vi "GenNewTraj.vi"(4 "MEGA traj":T1 {"?"."Limits"."StoopidFast (fps)" min=0.0; "?"."Limits"."Jerk (fps^3)" min=0.0 step=1.0; "?"."Limits"."Accel (fps^2)" min=0.0; "?"."Limits"."Velocity (fps)" min=0.0; "?"."Overrides"."Angle Override" step=5.0; "?"."Overrides"."Velocity Override" step=5.0; "?"."Overrides"."Angular Override" step=5.0; "?"."Angular Limits"."Jerk (deg/s^3)" min=0.0 step=1.0; "?"."Angular Limits"."Accel (deg/s^2)" min=0.0; "?"."Angular Limits"."Velocity (deg/s)" min=0.0}, 6 "Drive Type":T9, 7 "MEGA?":bool, 8 "Stoopid Overlap %":dbl min=0.0, 9 "Path Type":T10, 10 "Parameters":T11 {"Limits"."StoopidFast (fps)" min=0.0; "Limits"."Jerk (fps^3)" min=0.0 step=1.0; "Limits"."Accel (fps^2)" min=0.0; "Limits"."Velocity (fps)" min=0.0; "Overrides"."Angle Override" step=5.0; "Overrides"."Velocity Override" step=5.0; "Overrides"."Angular Override" step=5.0; "Angular Limits"."Jerk (deg/s^3)" min=0.0 step=1.0; "Angular Limits"."Accel (deg/s^2)" min=0.0; "Angular Limits"."Velocity (deg/s)" min=0.0}, 11 "Points in":cluster{"x":dbl, "y":dbl, "th":dbl}[](array[cluster])) -> (0 "Time & Dist":cluster{"Time (s)":dbl, "Distance (ft)":dbl}, 1 "Valid":bool, 2 "Trajectory Data":T2, 3 "Updated Waypoints":cluster{"x":dbl, "y":dbl, "th":dbl}[](array[cluster]), 5 "MEGA traj 2":T1 {"?"."Limits"."StoopidFast (fps)" min=0.0; "?"."Limits"."Jerk (fps^3)" min=0.0 step=1.0; "?"."Limits"."Accel (fps^2)" min=0.0; "?"."Limits"."Velocity (fps)" min=0.0; "?"."Overrides"."Angle Override" step=5.0; "?"."Overrides"."Velocity Override" step=5.0; "?"."Overrides"."Angular Override" step=5.0; "?"."Angular Limits"."Jerk (deg/s^3)" min=0.0 step=1.0; "?"."Angular Limits"."Accel (deg/s^2)" min=0.0; "?"."Angular Limits"."Velocity (deg/s)" min=0.0})   [LabVIEW 2023]
uses:
  Types/Trajectory Data.ctl
  Types/Segment Type.ctl
  Types/Path Type.ctl
  Types/Limits.ctl
  Types/Overrides.ctl
  Types/Angluar Limits.ctl
  Types/Drive Type.ctl
  FileIO/MEGA traj.ctl
  Types/Single Cmd Info.ctl
  <vilib>/picture/picture.llb/imagedata.ctl
  Bezier/Bezier Trajectory.vi
  Clothoid/Generate Clothoid Trajectory.vi
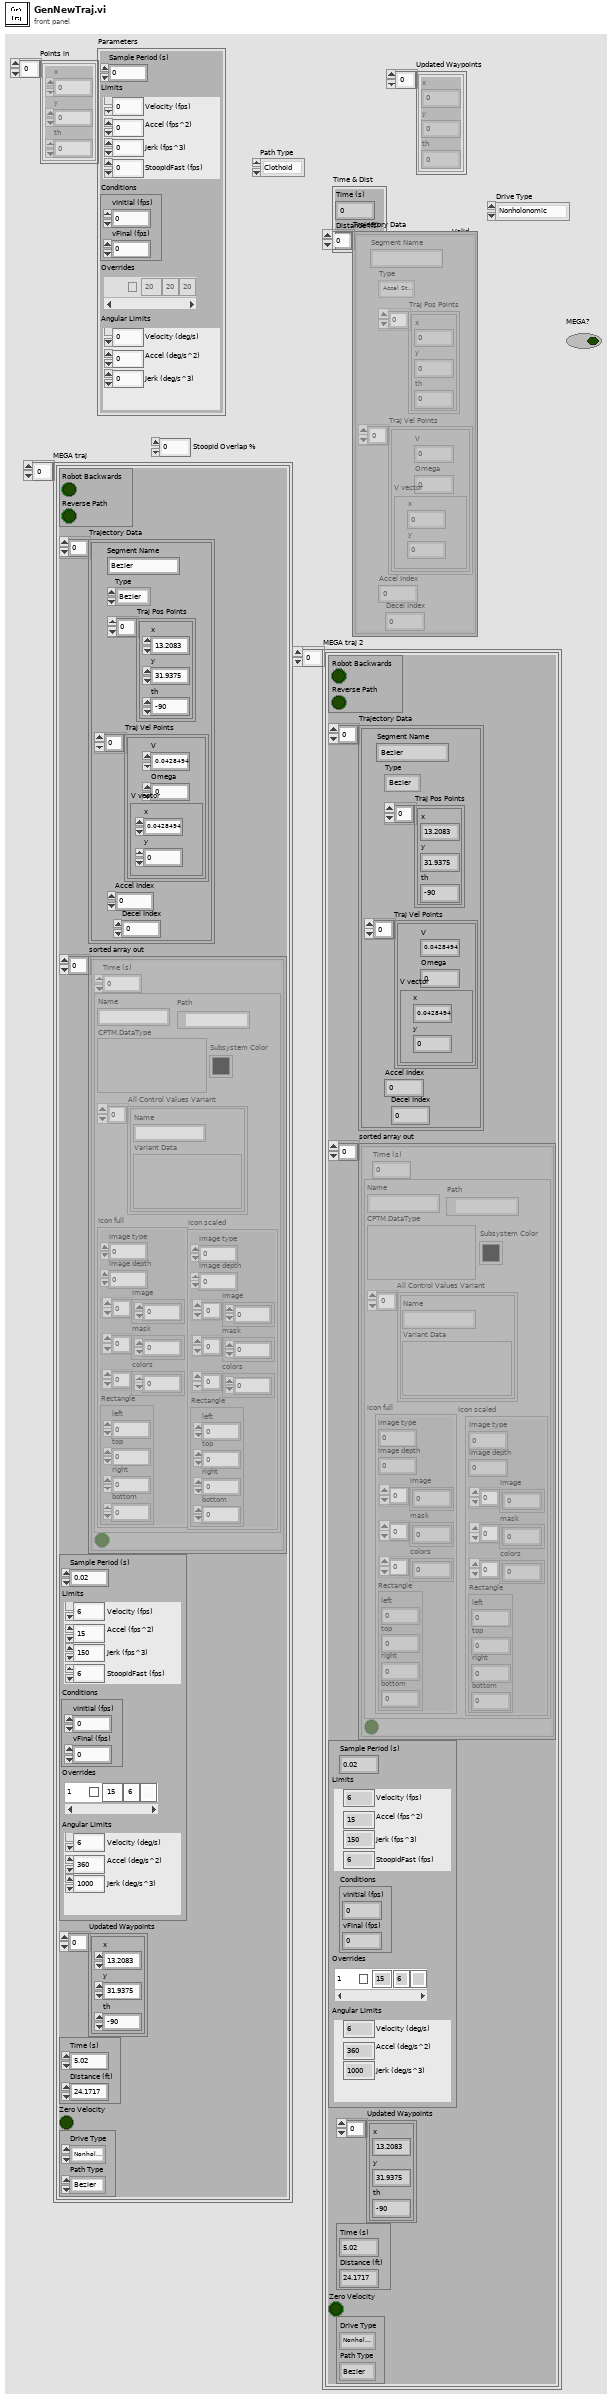
[diagram p1: front panel]
types:
  T1 = typedef "MEGA traj.ctl" = cluster{cluster{"Robot Backwards":bool, "Reverse Path":bool}, "Trajectory Data":T2, "sorted array out":cluster{"Time (s)":dbl, T4, bool}[], cluster{"Sample Period (s)":dbl, "Limits":T6, "Conditions":cluster{"vInitial (fps)":dbl, "vFinal (fps)":dbl}, "Overrides":T7, "Angular Limits":T8}, "Updated Waypoints":cluster{"x":dbl, "y":dbl, "th":dbl}[], cluster{"Time (s)":dbl, "Distance (ft)":dbl}, "Zero Velocity":bool, cluster{"Drive Type":T9, "Path Type":T10}}[]
  T2 = typedef "Trajectory Data.ctl" = cluster{"Segment Name":string, "Type":T3, "Traj Pos Points":cluster{"x":dbl, "y":dbl, "th":dbl}[], "Traj Vel Points":cluster{"V":dbl, "Omega":dbl, "V vector":cluster{"y":dbl, "x":dbl}}[], "Accel Index":i32, "Decel Index":i32}[]
  T3 = typedef "Segment Type.ctl" = enum16{"Accel Straight", "Const Straight", "Blend", "Circle", "Bezier"}
  T4 = typedef "Single Cmd Info.ctl" = cluster{"Name":string, "CPTM.DataType":variant, "All Control Values Variant":cluster{"Name":string, "Variant Data":variant}[], "icon full":T5, "icon scaled":T5, "Path":path, "Subsystem Color":u32}
  T5 = typedef "imagedata.ctl" = cluster{"image type":i32, "image depth":i32, "image":u8[], "mask":u8[], "colors":u32[], "Rectangle":cluster{"left":i16, "top":i16, "right":i16, "bottom":i16}}
  T6 = typedef "Limits.ctl" = cluster{"Velocity (fps)":dbl, "Accel (fps^2)":dbl, "Jerk (fps^3)":dbl, "StoopidFast (fps)":dbl}
  T7 = typedef "Overrides.ctl" = cluster{"Count":string, "Angular Override":dbl, "Enabled?":bool, "Velocity Override":dbl, "Angle Override":dbl}[]
  T8 = typedef "Angluar Limits.ctl" = cluster{"Velocity (deg/s)":dbl, "Accel (deg/s^2)":dbl, "Jerk (deg/s^3)":dbl}
  T9 = typedef "Drive Type.ctl" = enum16{"Nonholonomic", "Holonomic"}
  T10 = typedef "Path Type.ctl" = enum16{"Clothoid", "Bezier"}
  T11 = cluster{"Sample Period (s)":dbl, "Limits":T6, "Conditions":cluster{"vInitial (fps)":dbl, "vFinal (fps)":dbl}, "Overrides":T7, "Angular Limits":T8}
  T12 = cluster{"Robot Backwards":bool, "Reverse Path":bool}
  T13 = cluster{"vInitial (fps)":dbl, "vFinal (fps)":dbl}
  T14 = cluster{"Segment Name":string, "Type":T3, "Traj Pos Points":cluster{"x":dbl, "y":dbl, "th":dbl}[], "Traj Vel Points":cluster{"V":dbl, "Omega":dbl, "V vector":cluster{"y":dbl, "x":dbl}}[], "Accel Index":i32, "Decel Index":i32}[]
  T15 = cluster{cluster{"Robot Backwards":bool, "Reverse Path":bool}, "Trajectory Data":T2, "sorted array out":cluster{"Time (s)":dbl, T4, bool}[], cluster{"Sample Period (s)":dbl, "Limits":T6, "Conditions":cluster{"vInitial (fps)":dbl, "vFinal (fps)":dbl}, "Overrides":T7, "Angular Limits":T8}, "Updated Waypoints":cluster{"x":dbl, "y":dbl, "th":dbl}[], cluster{"Time (s)":dbl, "Distance (ft)":dbl}, "Zero Velocity":bool, cluster{"Drive Type":T9, "Path Type":T10}}
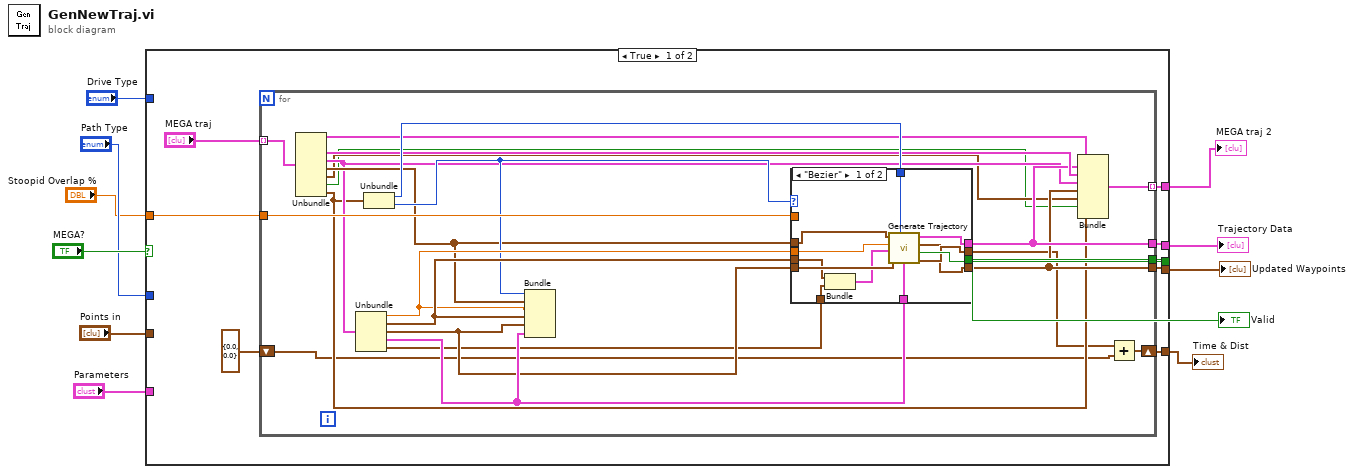
[diagram p0: block diagram]
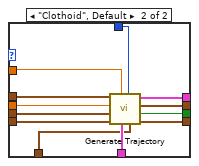
[diagram p2: hidden frame]
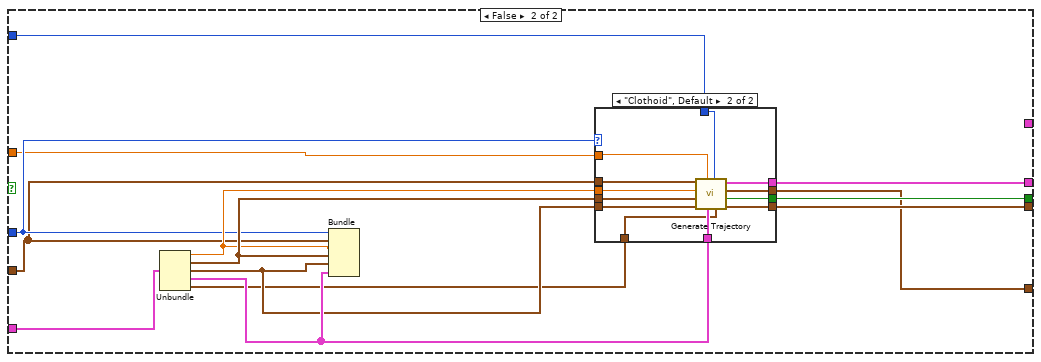
[diagram p3: hidden frame]
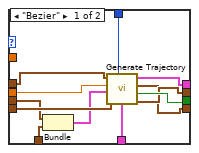
[diagram p4: hidden frame]
diagram:
  n1 = case shown="True" "MEGA?" {
    tunnel: [w17 w80] -> w11
    tunnel: [w16 w79] -> w10
    tunnel: [w18 w75] -> w9
    tunnel: [w19 w73] -> w8
    tunnel: "Drive Type" -> [_ w71]
    tunnel: "Path Type" -> [_ w70]
    tunnel: "Stoopid Overlap %" -> [w14 w69]
    tunnel: "Points in" -> [_ w68]
    tunnel: "Parameters" -> [_ w67]
    tunnel: [w13 _] -> w1
    frame True {
      n2 = for {
        tunnel: [w29] -> w19
        tunnel: [w37] -> w17
        tunnel: [w27] -> w16
        tunnel: w14 -> [w36]
        tunnel: "MEGA traj" -> [w35] mode=indexing
        tunnel: [w23] -> w13 mode=indexing
        shift-right: [w22] -> w18
        shift-left: cluster{"Time (s)":dbl, "Distance (ft)":dbl} {"Time (s)"=0.0, "Distance (ft)"=0.0} -> [w20]
        n3 = Unbundle(w35) -> (w31:T12, "sorted array out"=w30:cluster{"Time (s)":dbl, T4, bool}[], w28:T11, "Updated Waypoints"=w32:cluster{"x":dbl, "y":dbl, "th":dbl}[], w26:cluster{"Time (s)":dbl, "Distance (ft)":dbl}, "Zero Velocity"=w25:bool, w24:cluster{"Drive Type":T9, "Path Type":T10})  [unwired: 1 out]
        n4 = Unbundle(w28) -> ("Sample Period (s)"=w39:dbl, "Limits"=w41:T6, "Conditions"=w40:T13, "Overrides"=w42:T7, "Angular Limits"=w38:T8)
        n5 = Unbundle(w24) -> ("Drive Type"=w34:T9, "Path Type"=w33:T10)
        n6 = Bundle("Path Type"=w33, "Updated Waypoints"=w32, "Sample Period (s)"=w39, "Limits"=w41, "Conditions"=w40, "Overrides"=w42) -> ()  [unwired: 1 in, 1 out]
        n7 = case shown="\"Bezier\"" w33 {
          tunnel: [w51 w66] -> w37
          tunnel: [w49 w65] -> w21
          tunnel: w40 -> [w53 w64]
          tunnel: w41 -> [w45 w63]
          tunnel: w42 -> [w52 w62]
          tunnel: [w48 w61] -> w27
          tunnel: [w50 w56] -> w29
          tunnel: w36 -> [_ w60]
          tunnel: w32 -> [w54 w59]
          tunnel: w39 -> [w47 w58]
          tunnel: w34 -> [w46 w57]
          tunnel: w38 -> [w44 w55]
          frame "Bezier" {
            n8 = Bundle("Limits"=w45, "Angular Limits"=w44) -> (w43:cluster{"Limits":T6, "Angular Limits":T8})  [unwired: 1 in]
            n9 = call-poly "Generate Trajectory.vi"("Overrides"=w52, "Drive Type"=w46, "Conditions"=w53, "All Limits"=w43, "sample period (s)"=w47, "WayPoints"=w54) -> ("Time & Dist"=w49:cluster{"Time (s)":dbl, "Distance (ft)":dbl}, "Valid"=w51:bool, "Updated Waypoints"=w48:cluster{"x":dbl, "y":dbl, "th":dbl}[], "Trajectory Data"=w50:T2)  [unwired: 2 in]
          }
          frame "Clothoid", Default {
            n10 = call-poly "Generate Trajectory.vi"("Angular Limits"=w55, "Drive Type"=w57, "Overrides"=w62, "Stoopid Overlap %"=w60, "Conditions"=w64, "Limits"=w63, "Sample Period (s)"=w58, "WayPoints"=w59) -> ("Updated Waypoints"=w61:cluster{"x":dbl, "y":dbl, "th":dbl}[], "Valid"=w66:bool, "Time & Dist"=w65:cluster{"Time (s)":dbl, "Distance (ft)":dbl}, "Trajectory Data Out"=w56:T14)
          }
        }
        n11 = Bundle(w31, "Trajectory Data"=w29, "sorted array out"=w30, w28, "Updated Waypoints"=w27, w26, "Zero Velocity"=w25, w24) -> (w23:T15)  [unwired: 1 in]
        n12 = Add(x=w21, y=w20) -> (x+y=w22:cluster{"Time (s)":dbl, "Distance (ft)":dbl})
      }
    }
    frame False {
      n13 = Unbundle(w67) -> ("Sample Period (s)"=w74:dbl, "Limits"=w77:T6, "Conditions"=w76:T13, "Overrides"=w78:T7, "Angular Limits"=w72:T8)
      n14 = Bundle("Path Type"=w70, "Points in"=w68, "Sample Period (s)"=w74, "Limits"=w77, "Conditions"=w76, "Overrides"=w78) -> ()  [unwired: 1 in, 1 out]
      n15 = case shown="\"Clothoid\", Default" w70 {
        tunnel: [w89 w104] -> w80
        tunnel: [w87 w103] -> w75
        tunnel: w76 -> [w91 w102]
        tunnel: w77 -> [w83 w101]
        tunnel: w78 -> [w90 w100]
        tunnel: [w86 w99] -> w79
        tunnel: [w88 w94] -> w73
        tunnel: w69 -> [_ w98]
        tunnel: w68 -> [w92 w97]
        tunnel: w74 -> [w85 w96]
        tunnel: w71 -> [w84 w95]
        tunnel: w72 -> [w82 w93]
        frame "Bezier" {
          n16 = Bundle("Limits"=w83, "Angular Limits"=w82) -> (w81:cluster{"Limits":T6, "Angular Limits":T8})  [unwired: 1 in]
          n17 = call-poly "Generate Trajectory.vi"("Overrides"=w90, "Drive Type"=w84, "Conditions"=w91, "All Limits"=w81, "sample period (s)"=w85, "WayPoints"=w92) -> ("Time & Dist"=w87:cluster{"Time (s)":dbl, "Distance (ft)":dbl}, "Valid"=w89:bool, "Updated Waypoints"=w86:cluster{"x":dbl, "y":dbl, "th":dbl}[], "Trajectory Data"=w88:T2)  [unwired: 2 in]
        }
        frame "Clothoid", Default {
          n18 = call-poly "Generate Trajectory.vi"("Angular Limits"=w93, "Drive Type"=w95, "Overrides"=w100, "Stoopid Overlap %"=w98, "Conditions"=w102, "Limits"=w101, "Sample Period (s)"=w96, "WayPoints"=w97) -> ("Updated Waypoints"=w99:cluster{"x":dbl, "y":dbl, "th":dbl}[], "Valid"=w104:bool, "Time & Dist"=w103:cluster{"Time (s)":dbl, "Distance (ft)":dbl}, "Trajectory Data Out"=w94:T14)
        }
      }
    }
  }
  "Valid" <- w11
  "Updated Waypoints" <- w10
  "Time & Dist" <- w9
  "Trajectory Data" <- w8
  "MEGA traj 2" <- w1
